vi "Reset DMM.vi"(8 "error in (no error)":errorcluster, 10 "Reset Scope":string, 11 "VISA resource name":refnum<visa-resource-name>) -> (0 "error out":errorcluster, 2 "Command String":string, 3 "VISA resource name out":refnum<visa-resource-name>)   [LabVIEW 2018, in "Keithley 3706.lvlib"]
uses:
  <instrlib>/Keithley 3706/Keithley 3706.lvlib
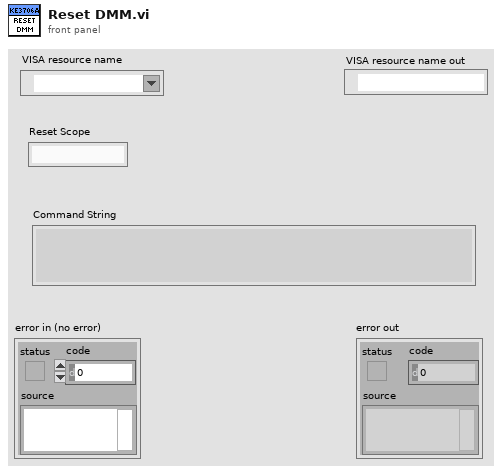
[diagram p1: front panel]
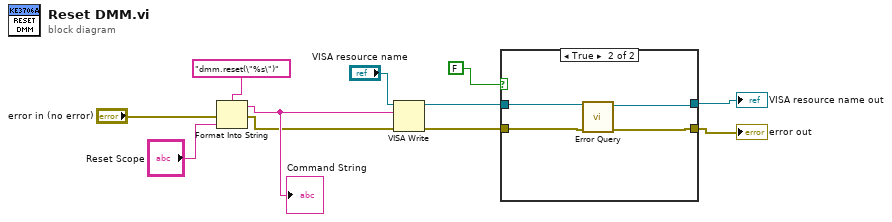
[diagram p0: block diagram]
diagram:
  n1 = Format Into String(format string="dmm.reset(\"%s\")", error in="error in (no error)", "Reset Scope") -> (resulting string=w7:string, error out=w6:errorcluster)  [unwired: 1 in]
  "Command String" <- w7
  n2 = VISA Write(VISA resource name="VISA resource name", write buffer=w7, error in (no error)=w6) -> (VISA resource name out=w4:refnum<visa-resource-name>, error out=w3:errorcluster)  [unwired: 1 out]
  n3 = case shown="True" FALSE {
    tunnel: w4 -> [w13 w17]
    tunnel: w3 -> [w12 w16]
    tunnel: [w13 w15] -> w1
    tunnel: [w12 w14] -> w2
    frame False {
    }
    frame True {
      n4 = call <instrlib>:"Error Query.vi"("error in (no error)"=w16, "VISA resource name"=w17) -> ("error out"=w14:errorcluster, "VISA resource name output"=w15:refnum<visa-resource-name>)  [unwired: 6 in, 2 out]
    }
  }
  "VISA resource name out" <- w1
  "error out" <- w2
